vi "UHR-Fleezers Control (host) - 11.1.vi"() -> ()   [LabVIEW 2012] (continued)
            n1098 = Divide(x=w2503, y=w2487) -> (x/y=w2502:dbl[])
            n1099 = Build Array(w2522, w2521, w2536, w2520, w2519, w2533, w2488, w2504, w2489, w2486, w2502, w2487, w2500, w2499) -> (w2498:dbl[][])
            n1100 = Bundle("T1 Y", "T1 X", "T1 Sum", "T2 Y", "T2 X", "T2 Sum", "T1 FB Y", "T1 FB X", "T1 FB Sum", "T2 FB Y", "T2 FB X", "T2 FB Sum", "PSD X", "PSD Y Sum") -> (w2485:T40)  [unwired: 1 out]
            n1101 = To Word Integer(number=w2540) -> (16bit integer=w2484:i16[])
            n1102 = Cluster To Array(cluster=w2485) -> (array=w2531:string[])
          }
        }
      }
    }
    "AI labels" <- w1617
    n1103 = Decimate 1D Array(w1591) -> (w1615:void[], w1559:void[])
    n1104 = local read "DMA Update Period (s)"() -> (w1627:dbl)
    n1105 = Build Array(w1615, w1559) -> (w1693:void[])
    n1106 = local read "Data Period (s)"() -> (w1465:dbl)
    n1107 = local read "BD 1 Frequency 2 (MHz)"() -> (w1498:dbl)
    n1108 = local read "BD 1 Frequency 1 (MHz)"() -> (w1499:dbl)
    n1109 = Decimate 1D Array(w1506) -> (w1530:i16[], w1529:i16[], w1527:i16[], w1526:i16[])  [unwired: 9 out]
    n1110 = To Double Precision Float(number=w1693) -> (double precision float=w1694:dbl[])
    n1111 = local read "APD Integration Time (s)"() -> (w1572:dbl)
    n1112 = Multiply(x=w1465, y="Trap Pos. Disp. Downsample") -> (x*y=w1463:dbl)
    n1113 = Divide(x=w1530, y=w1529) -> (x/y=w1531:dbl[])
    n1114 = Divide(x=w1527, y=w1526) -> (x/y=w1528:dbl[])
    n1115 = feedback #6(0.0) -> (w1544:dbl)
    n1116 = Add(x=w1627, y=w1544) -> (x+y=w1733:dbl)
    n1117 = feedback-in #6(w1733) -> ()
    n1118 = local read "AOM X Cal (nm/MHz)"() -> (w1496:dbl)
    n1119 = To Time Stamp(1:w1544) -> (0:w1543:timestamp)
    n1120 = Split 1D Array(array=w1531, index="N El. to Ave.") -> (second subarray=w1534:dbl[])  [unwired: 1 out]
    n1121 = Split 1D Array(array=w1528, index="N El. to Ave.") -> (second subarray=w1533:dbl[])  [unwired: 1 out]
    n1122 = Multiply(x=w1465, y="Trap Disp. Downsample") -> (x*y=w1545:dbl)
    "Display Period (s)" <- w1545
    n1123 = for "Trap AI" {
      tunnel: [w2283] -> w1727 mode=indexing
      tunnel: w1543 -> [w2273]
      tunnel: "Trap Disp. Downsample" -> [w2281]
      tunnel: w1618 -> [w2279] mode=indexing
      tunnel: w1465 -> [w2278]
      tunnel: w1617 -> [w2277] mode=indexing
      tunnel: w1542 -> [w2276]
      tunnel: [w2275] -> w1583 mode=indexing
      tunnel: w1545 -> [w2274]
      workers-P: _ -> [_]
      n1124 = Bundle By Name("Y"=w2279, "dt"=w2278) -> (w2280:waveform(dbl))  [unwired: 1 out]
      n1125 = Set Waveform Attribute(5:w2277, 6:w2276, 7:w2280) -> (3:w2275:waveform(dbl))  [unwired: 1 in, 2 out]
      n1126 = call "downsample 1D array - double.vi"("Ave N"=w2281, "Array In"=w2279) -> ("Array Out"=w2282:dbl[])  [unwired: 1 out]
      n1127 = Bundle By Name(cluster=w2275, "t0"=w2273, "Y"=w2282, "dt"=w2274) -> (w2283:waveform(dbl))
    }
    n1128 = Bundle("BD 1 Frequency 1 (MHz)"=w1499, "BD 1 Frequency 2 (MHz)"=w1498) -> (w1500:T41)  [unwired: 1 out]
    n1129 = call-poly <vilib>:"Mean.vi"("X"=w1533) -> ("mean"=w1521:dbl)  [unwired: 1 out]
    n1130 = call-poly <vilib>:"Mean.vi"("X"=w1534) -> ("mean"=w1522:dbl)  [unwired: 1 out]
    n1131 = Reciprocal(x=w1545) -> (1/x=→"Trap Disp. Freq. (Hz)":dbl)
    n1132 = Cluster To Array(cluster=w1500) -> (array=w1497:dbl[])
    n1133 = local read "Trap X AI1 (DMA)"() -> (w1532:T13)
    n1134 = local read "Data points/scans (MCL)"() -> (w1705:dbl)
    n1135 = To Fixed-Point(number=w1521) -> (fixed-point=w1519:fxp<+/-,16,1>)  [unwired: 1 in]
    n1136 = To Fixed-Point(number=w1522) -> (fixed-point=w1520:fxp<+/-,16,1>)  [unwired: 1 in]
    n1137 = Bundle("Trap 1 Pos.", "Trap 2 Pos.") -> (w1541:cluster{string, string})  [unwired: 1 out]
    n1138 = Bundle By Name(cluster=w1532, "Set 1"=w1520, "Set 2"=w1519) -> (→"Trap X AI1 (DMA)":T13)
    n1139 = Cluster To Array(cluster=w1541) -> (array=w1538:string[])
    n1140 = Bundle("APD 1", "APD 2") -> (w1726:cluster{string, string})  [unwired: 1 out]
    n1141 = Select(t=-1.0, s="Negate Y Axis", f=1.0) -> (s? t:f=w1482:dbl)
    n1142 = for "Trap Position" {
      tunnel: w1547 -> [w1922] mode=indexing
      tunnel: "Trap Pos. Disp. Downsample" -> [w1921]
      tunnel: w1463 -> [w1919]
      tunnel: w1543 -> [w1918]
      tunnel: w1542 -> [w1916]
      tunnel: w1538 -> [w1915] mode=indexing
      tunnel: [w1914] -> w1452 mode=indexing
      tunnel: w1497 -> [w1912] mode=indexing
      tunnel: w1496 -> [w1910]
      tunnel: w1482 -> [w1909]
      n1143 = call "downsample 1D array - double.vi"("Ave N"=w1921, "Array In"=w1922) -> ("Array Out"=w1920:dbl[])  [unwired: 1 out]
      n1144 = Subtract(x=w1920, y=w1912) -> (x-y=w1913:dbl[])
      n1145 = Multiply(x=w1910, y=w1913) -> (x*y=w1911:dbl[])
      n1146 = Multiply(x=w1909, y=w1911) -> (x*y=w1908:dbl[])
      n1147 = Bundle By Name("Y"=w1908, "dt"=w1919, "t0"=w1918) -> (w1917:waveform(dbl))  [unwired: 1 out]
      n1148 = Set Waveform Attribute(5:w1915, 6:w1916, 7:w1917) -> (3:w1914:waveform(dbl))  [unwired: 1 in, 2 out]
    }
    n1149 = Cluster To Array(cluster=w1726) -> (array=w1723:string[])
    n1150 = for "APD" {
      tunnel: w1694 -> [w2262] mode=indexing
      tunnel: w1572 -> [w2270]
      tunnel: [w2266] -> w1579 mode=indexing
      tunnel: "APD Disp. Scale" -> [w2267]
      tunnel: w1542 -> [w2265]
      tunnel: w1723 -> [w2264] mode=indexing
      tunnel: "APD Disp. Downsample" -> [w2260]
      tunnel: [w2263] -> w1722
      workers-P: _ -> [_]
      tunnel: w1543 -> [w2259]
      n1151 = call "integrate 1D array interval - double.vi"("Ave N"=w2260, "Array In"=w2262) -> ("Array Out"=w2261:dbl[])  [unwired: 1 out]
      n1152 = Multiply(x=w2270, y=w2260) -> (x*y=w2263:dbl)
      n1153 = Divide(x=w2261, y=w2267) -> (x/y=w2268:dbl[])
      n1154 = Bundle By Name("t0"=w2259, "Y"=w2268, "dt"=w2263) -> (w2269:waveform(dbl))  [unwired: 1 out]
      n1155 = Set Waveform Attribute(5:w2264, 6:w2265, 7:w2269) -> (3:w2266:waveform(dbl))  [unwired: 1 in, 2 out]
    }
    "APD Display Period (s)" <- w1722
    n1156 = Reciprocal(x=w1722) -> (1/x=→"APD Display Freq. (Hz)":dbl)
    n1157 = local read "Display Period (s)"() -> (w1603:dbl)
    n1158 = Increment(x=w1705) -> (x+1=w1706:dbl)
    n1159 = To Double Precision Float(number=w1615) -> (double precision float=w1614:dbl[])
    n1160 = Index Array(array=w1452, index=0) -> (element=w1456:waveform(dbl))
    n1161 = Index Array(array=w1452, index=1) -> (element=w1451:waveform(dbl))
    n1162 = feedback #7(w1706) -> (w1709:dbl)
    n1163 = Select(t=0, s=w1696, f=w1709) -> (s? t:f=w1702:dbl)
    n1164 = Array Size(array=w1614) -> (size(s)=w1708:i32)
    n1165 = Add(x=w1708, y=w1702) -> (x+y=w1703:dbl)
    n1166 = Unbundle By Name(w1456) -> ("Y"=w1457:dbl[])
    n1167 = feedback #8(w1615) -> (w1692:void[])
    n1168 = Build Array (concatenate)(w1692, w1615) -> (w1689:void[])
    n1169 = feedback #9(w1559) -> (w1578:void[])
    n1170 = Divide(x="Bead Sep. Int. Time (s)", y=w1603) -> (x/y=w1492:dbl)
    n1171 = Build Array (concatenate)(w1578, w1559) -> (w1577:void[])
    n1172 = Add(x=w1457, y="FB Trap Pos Offset") -> (x+y=w1455:dbl[])
    "T1 x pos data" <- w1455
    n1173 = Greater?(x=w1703, y=w1705) -> (0:w1704:bool)
    n1174 = feedback #10(w1455) -> (w1494:dbl[])
    n1175 = Build Array (concatenate)(w1455, w1494) -> (w1493:dbl[])
    n1176 = Bundle By Name(cluster=w1456, "Y"=w1455) -> (w1454:waveform(dbl))
    n1177 = Select(t=w1702, s=w1704, f=w1703) -> (s? t:f=w1701:dbl)
    n1178 = feedback-in #7(w1701) -> ()
    n1179 = Array Size(array=w1689) -> (size(s)=w1686:i32)
    n1180 = Array Size(array=w1615) -> (size(s)=w1688:i32)
    n1181 = local read "MCL Scanning"() -> (w1699:bool)
    n1182 = local read "APD Integration Time (s)"() -> (w1586:dbl)
    n1183 = Bundle(w1454, w1451) -> (w1450:cluster{waveform(dbl), waveform(dbl)})  [unwired: 1 out]
    n1184 = Build Array (concatenate)(w1579, w1727) -> (w1581:waveform(dbl)[])
    "All Signals" <- w1581
    n1185 = Split 1D Array(array=w1493, index=w1492) -> (first subarray=w1486:dbl[])  [unwired: 1 out]
    n1186 = feedback-in #10(w1486) -> ()
    n1187 = Multiply(x=w1688, y="APD Ave N") -> (x*y=w1687:dbl)
    n1188 = Greater?(x=w1686, y=w1687) -> (0:w1690:bool)
    n1189 = Not(x=w1704) -> (.not. x?=w1698:bool)
    n1190 = Cluster To Array(cluster=w1450) -> (array=w1426:waveform(dbl)[])
    "Trap Positions" <- w1426
    n1191 = To Double Precision Float(number=w1559) -> (double precision float=w1558:dbl[])
    n1192 = call-poly <vilib>:"Mean.vi"("X"=w1486) -> ("mean"=w1485:dbl)  [unwired: 1 out]
    "Mean T1 Position (nm)" <- w1485
    n1193 = Subtract(x=w1486, y=w1485) -> (x-y=w1491:dbl[])
    n1194 = Square(x=w1491) -> (x^2=w1490:dbl[])
    n1195 = And(x=w1698, y=w1699) -> (x .and. y?=w1700:bool)
    n1196 = call-poly <vilib>:"Mean.vi"("X"=w1490) -> ("mean"=w1489:dbl)  [unwired: 1 out]
    n1197 = case shown="True" w1690 {
      tunnel: w1689 -> [w2042 w2049]
      tunnel: [w2042 w2047] -> w1632
      tunnel: w1687 -> [_ w2044]
      tunnel: w1686 -> [_ w2048]
      tunnel: w1577 -> [w2041 w2046]
      tunnel: [w2041 w2043] -> w1574
      frame False {
      }
      frame True {
        n1198 = Subtract(x=w2048, y=w2044) -> (x-y=w2045:dbl)
        n1199 = Array Subset(array=w2049, index=w2045, length=w2044) -> (w2047:void[])
        n1200 = Array Subset(array=w2046, index=w2045, length=w2044) -> (w2043:void[])
      }
    }
    n1201 = feedback-in #8(w1632) -> ()
    n1202 = feedback-in #9(w1574) -> ()
    n1203 = Square Root(x=w1489) -> (sqrt(x)=w1488:dbl)
    n1204 = Or(x=w1700, y=w1696) -> (x .or. y?=w1697:bool)
    n1205 = Equal?(x="Tab Control 6", y=T29."High Res Display") -> (x = y?=w1621:bool)
    n1206 = Multiply(x="APD Disp. Scale", y=w1579) -> (x*y=w1588:waveform(dbl)[])
    n1207 = Multiply(x=10.0, y=w1488) -> (x*y=→"Trap 1 Position RMS (A)":dbl)
    n1208 = Multiply(x="APD Disp. Downsample", y=w1586) -> (x*y=w1584:dbl)
    n1209 = Divide(x=w1588, y=w1584) -> (x/y=w1556:waveform(dbl)[])
    n1210 = case "For displaying the high resolution display (no downsampling)" shown="True" w1621 {
      tunnel: w1583 -> [_ w1942]
      frame False {
      }
      frame True {
        n1211 = Index Array(array=w1942, index="High Res. Display") -> (element=w1943:waveform(dbl))
        n1212 = call <vilib>:"Std Deviation and Variance.vi"("X"=w1943) -> ("mean"=w1950:dbl, "standard deviation"=w1955:dbl)  [unwired: 1 in, 1 out]
        "Mean Intensity" <- w1950
        "Sigma" <- w1955
        n1213 = Subtract(x=w1943, y=w1950) -> (x-y=w1949:waveform(dbl))
        n1214 = Select(t=w1949, s="Subtract mean", f=w1943) -> (s? t:f=→"1 Channel":waveform(dbl))
        n1215 = Divide(x=w1955, y=w1950) -> (x/y=→"Sigma/Mean":dbl)
        n1216 = feedback #11(1) -> (w1944:i32)
        n1217 = Greater Or Equal?(x=w1944, y="Slow mean N ave.") -> (x >= y?=w1957:bool)
        n1218 = Increment(x=w1944) -> (x+1=w1959:i32)
        n1219 = Select(t=1, s=w1957, f=w1959) -> (s? t:f=w1946:i32)
        n1220 = feedback-in #11(w1946) -> ()
        n1221 = feedback #12() -> (w1947:waveform(dbl))  [unwired: 1 out]
        n1222 = case shown="Default" w1944 {
          tunnel: [w1962 w1965] -> w1948
          tunnel: w1947 -> [w1964 _]
          tunnel: w1943 -> [w1963 w1965]
          frame Default {
            n1223 = call-poly <vilib>:"Append Waveforms.vi"("waveform B"=w1963, "waveform A"=w1964) -> ("waveform out"=w1962:waveform(dbl))  [unwired: 1 in, 8 out]
          }
          frame 1 {
          }
        }
        n1224 = feedback-in #12(w1948) -> ()
        n1225 = case shown="True" w1957 {
          tunnel: w1948 -> [_ w1961]
          frame False {
          }
          frame True {
            n1226 = call-poly <vilib>:"Mean.vi"("X"=w1961) -> ("mean"=→"Slow mean":dbl)  [unwired: 1 out]
          }
        }
      }
    }
    n1227 = Index Array(array=w1556, index=0) -> (element=w1566:waveform(dbl))
    n1228 = Index Array(array=w1556, index=1) -> (element=w1564:waveform(dbl))
    n1229 = case "For computing FFTs for display" shown="True" "Compute FFT" {
      tunnel: w1583 -> [_ w2656]
      frame False {
      }
      frame True {
        n1230 = Build Array("FFT 1 Choice 1", "FFT 1 Choice 2", "FFT 2 Choice 1", "FFT 2 Choice 2") -> (w2649:u16[])
        n1231 = Array Size(array=w2656) -> (size(s)=w2655:i32)
        n1232 = feedback-in #13(w2649) -> ()
        n1233 = feedback #13(u16[] [100, 100, 100, 100]) -> (w2650:u16[])
        n1234 = feedback-in #14("# Spectra to Ave.") -> ()
        n1235 = feedback #14("# Spectra to Ave.") -> (w2647:dbl)
        n1236 = Not Equal?(x="# Spectra to Ave.", y=w2647) -> (x != y?=w2646:bool)
        n1237 = Not Equal?(x=w2649, y=w2650) -> (x != y?=w2648:bool)
        n1238 = feedback #15(1.0) -> (w2633:dbl)
        n1239 = Compound Arithmetic op=OR("Reset FFT", w2648, w2646) -> (w2631:bool)
        n1240 = Select(t=1.0, s=w2631, f=w2633) -> (s? t:f=w2635:dbl)
        n1241 = Greater?(x=w2635, y="# Spectra to Ave.") -> (0:w2654:bool)
        n1242 = Increment(x=w2635) -> (x+1=w2634:dbl)
        n1243 = feedback-in #15(w2634) -> ()
        n1244 = local read "DMA Update Period (s)"() -> (w2629:dbl)
        n1245 = Multiply(x="# Spectra to Ave.", y=w2629) -> (x*y=→"Ave. Time (s)":dbl)
        n1246 = Build Array(cluster{"f0":dbl, "df":dbl, "magnitude":dbl[]} {"f0"=0.0, "df"=0.0, "magnitude"=[]} ("PSD")) -> (w2638:cluster{"f0":dbl, "df":dbl, "magnitude":dbl[]}[])
        n1247 = Build Array(w2638, w2638, w2638, w2638) -> (w2640:T42)
        n1248 = feedback #16(w2640) -> (w2645:T42)
        n1249 = for {
          N: 4 -> [_]
          tunnel: w2649 -> [w2678] mode=indexing
          tunnel: w2656 -> [w2679]
          tunnel: w2655 -> [w2681]
          tunnel: w2631 -> [w2674]
          tunnel: w2654 -> [w2673]
          tunnel: "# Spectra to Ave." -> [w2672]
          tunnel: [w2671] -> w2644 mode=indexing
          tunnel: w2645 -> [w2676] mode=indexing
          tunnel: [w2675] -> w2632 mode=indexing
          tunnel: w2635 -> [w2670]
          n1250 = Less?(x=w2678, y=w2681) -> (x < y?=w2680:bool)
          n1251 = Index Array(array=w2679, index=w2678) -> (element=w2677:waveform(dbl))
          n1252 = case shown="True" w2680 {
            tunnel: w2677 -> [_ w2698]
            tunnel: w2676 -> [w2683 w2696]
            tunnel: [w2683 w2684] -> w2675
            tunnel: w2674 -> [_ w2695]
            tunnel: w2673 -> [_ w2688]
            tunnel: w2672 -> [_ w2687]
            tunnel: [cluster{"f0":dbl, "df":dbl, "magnitude":dbl[]} {"f0"=0.0, "df"=0.0, "magnitude"=[]} ("PSD") w2689] -> w2671
            tunnel: w2670 -> [_ w2686]
            frame False {
            }
            frame True {
              n1253 = call <vilib>:"Std Deviation and Variance.vi"("X"=w2698) -> ("mean"=w2699:dbl)  [unwired: 1 in, 2 out]
              n1254 = Subtract(x=w2698, y=w2699) -> (x-y=w2697:waveform(dbl))
              n1255 = xnode "Spectral Measurements"("Signals"=w2697) -> ("PSD"=w2691:cluster{"f0":dbl, "df":dbl, "magnitude":dbl[]})  [unwired: 1 in, 1 out]
              n1256 = case shown="False" w2695 {
                tunnel: w2696 -> [w2708 _]
                tunnel: [w2704 w2713] -> w2684
                tunnel: w2691 -> [w2707 w2714]
                tunnel: w2688 -> [w2706 _]
                frame False {
                  n1257 = Build Array (concatenate)(w2708, w2707) -> (w2705:cluster{"f0":dbl, "df":dbl, "magnitude":dbl[]}[])
                  n1258 = case shown="True" w2706 {
                    tunnel: w2705 -> [w2709 w2712]
                    tunnel: [w2709 w2710] -> w2704
                    frame False {
                    }
                    frame True {
                      n1259 = Delete From Array(array=w2712, index=0) -> (array with subset deleted=w2710:cluster{"f0":dbl, "df":dbl, "magnitude":dbl[]}[])  [unwired: 1 in, 1 out]
                    }
                  }
                }
                frame True {
                  n1260 = Build Array(w2714) -> (w2713:cluster{"f0":dbl, "df":dbl, "magnitude":dbl[]}[])
                }
              }
              n1261 = for {
                tunnel: w2684 -> [w2703] mode=indexing
                tunnel: [w2702] -> w2694 mode=indexing
                workers-P: _ -> [_]
                n1262 = Unbundle By Name(w2703) -> ("magnitude"=w2702:dbl[])
              }
              n1263 = Transpose 2D Array(2D array=w2694) -> (transposed array=w2693:dbl[][])
              n1264 = for {
                tunnel: w2693 -> [w2701] mode=indexing
                tunnel: [w2700] -> w2692 mode=indexing
                workers-P: _ -> [_]
                n1265 = Add Array Elements(numeric array=w2701) -> (sum=w2700:dbl)
              }
              n1266 = Select(t=w2687, s=w2688, f=w2686) -> (s? t:f=w2685:dbl)
              n1267 = Divide(x=w2692, y=w2685) -> (x/y=w2690:dbl[])
              n1268 = Bundle By Name(cluster=w2691, "magnitude"=w2690) -> (w2689:cluster{"f0":dbl, "df":dbl, "magnitude":dbl[]})
            }
          }
        }
        n1269 = case shown="True" w2631 {
          tunnel: w2632 -> [w2663 w2669]
          tunnel: [w2663 w2664] -> w2630
          frame False {
          }
          frame True {
            n1270 = Array Subset(array=w2669, index (row)=0 ("index"), length (row)=4 ("length"), index (col)=0 ("index"), length (col)=1 ("length")) -> (w2664:T42)
          }
        }
        n1271 = feedback-in #16(w2630) -> ()
        n1272 = Split 1D Array(array=w2644, index=2) -> (first subarray=→"FFT 1":cluster{"f0":dbl, "df":dbl, "magnitude":dbl[]}[], second subarray=→"FFT 2":cluster{"f0":dbl, "df":dbl, "magnitude":dbl[]}[])
      }
    }
    n1273 = case "For plotting results of scanning MCL" shown="True" w1697 {
      tunnel: w1696 -> [_ w2082]
      tunnel: w1614 -> [_ w2178]
      tunnel: w1705 -> [_ _]
      tunnel: w1583 -> [_ w2152]
      tunnel: w1558 -> [_ w2083]
      tunnel: w1557 -> [_ w2056]
      frame False {
      }
      frame True {
        w2063 = u32 0 items=["Horizontal", "Vertical", "Central", "1st Diagonal", "2nd Diagonal"] ("Type of Symmetry")
        w2091 = u32 0 items=["Horizontal", "Vertical", "Central", "1st Diagonal", "2nd Diagonal"] ("Type of Symmetry")
        w2094 = u32 0 items=["Horizontal", "Vertical", "Central", "1st Diagonal", "2nd Diagonal"] ("Type of Symmetry")
        w2123 = u32 0 items=["Horizontal", "Vertical", "Central", "1st Diagonal", "2nd Diagonal"] ("Type of Symmetry")
        n1274 = Index Array(array=w2152, index=10) -> (element=w2158:waveform(dbl))
        n1275 = Index Array(array=w2152, index=11) -> (element=w2155:waveform(dbl))
        n1276 = local read "Cycles/step (MCL)"() -> (w2108:u64)
        n1277 = Index Array(array=w2152, index="Channel") -> (element=w2154:waveform(dbl))
        n1278 = Unbundle(w2056) -> ("New Image"=w2055:T2, "New Image"=w2054:T2, "New Image"=w2053:T2, "New Image"=w2052:T2)
        n1279 = Unbundle By Name(w2158) -> ("Y"=w2110:dbl[])
        n1280 = Unbundle By Name(w2155) -> ("Y"=w2112:dbl[])
        n1281 = Unbundle By Name(w2154) -> ("Y"=w2117:dbl[])
        n1282 = call "downsample 1D array - double.vi"("Ave N"=w2108, "Array In"=w2110) -> ("Array Out"=w2109:dbl[])  [unwired: 1 out]
        n1283 = call "downsample 1D array - double.vi"("Ave N"=w2108, "Array In"=w2112) -> ("Array Out"=w2111:dbl[])  [unwired: 1 out]
        n1284 = call "downsample 1D array - double.vi"("Ave N"=w2108, "Array In"=w2117) -> ("Array Out"=w2116:dbl[])  [unwired: 1 out]
        n1285 = feedback #17(w2178) -> (w2179:dbl[])
        n1286 = Build Array (concatenate)(w2179, w2178) -> (w2160:dbl[])
        n1287 = feedback #18(w2083) -> (w2085:dbl[])
        n1288 = Build Array (concatenate)(w2085, w2083) -> (w2084:dbl[])
        n1289 = local read "Scan steps (MCL)"() -> (w2065:u64)
        n1290 = Select(t=w2178, s=w2082, f=w2160) -> (s? t:f=w2164:dbl[])
        n1291 = feedback-in #17(w2164) -> ()
        n1292 = Select(t=w2083, s=w2082, f=w2084) -> (s? t:f=w2066:dbl[])
        n1293 = feedback-in #18(w2066) -> ()
        n1294 = local read "Scan lines (y)"() -> (w2051:u64)
        n1295 = local read "N APD Samp/step"() -> (w2067:dbl)
        n1296 = feedback #19(w2109) -> (w2166:dbl[])
        n1297 = Build Array (concatenate)(w2166, w2109) -> (w2157:dbl[])
        n1298 = feedback #20(w2116) -> (w2176:dbl[])
        n1299 = Build Array (concatenate)(w2176, w2116) -> (w2175:dbl[])
        n1300 = feedback #21(w2111) -> (w2168:dbl[])
        n1301 = Build Array (concatenate)(w2168, w2111) -> (w2169:dbl[])
        n1302 = Select(t=w2109, s=w2082, f=w2157) -> (s? t:f=w2113:dbl[])
        n1303 = feedback-in #19(w2113) -> ()
        n1304 = Select(t=w2116, s=w2082, f=w2175) -> (s? t:f=w2115:dbl[])
        n1305 = feedback-in #20(w2115) -> ()
        n1306 = Select(t=w2111, s=w2082, f=w2169) -> (s? t:f=w2114:dbl[])
        n1307 = feedback-in #21(w2114) -> ()
        n1308 = Multiply(x=w2065, y=u64 2) -> (x*y=w2050:u64)
        n1309 = call "integrate 1D array interval - double.vi"("Ave N"=w2067, "Array In"=w2066) -> ("Array Out"=w2078:dbl[])  [unwired: 1 out]
        n1310 = call "integrate 1D array interval - double.vi"("Ave N"=w2067, "Array In"=w2164) -> ("Array Out"=w2163:dbl[])  [unwired: 1 out]
        n1311 = Array Size(array=w2078) -> (size(s)=w2079:i32)
        n1312 = Array Size(array=w2163) -> (size(s)=w2165:i32)
        n1313 = Multiply(x=w2051, y=w2050) -> (x*y=w2081:u64)
        n1314 = Multiply(x=w2051, y=w2050) -> (x*y=w2173:u64)
        n1315 = call-poly <vilib>:"Mean.vi"("X"=w2113) -> ("mean"=w2097:dbl)  [unwired: 1 out]
        n1316 = Subtract(x=w2081, y=w2079) -> (x-y=w2072:u64)
        n1317 = call-poly <vilib>:"Mean.vi"("X"=w2115) -> ("mean"=w2102:dbl)  [unwired: 1 out]
        n1318 = call-poly <vilib>:"Mean.vi"("X"=w2114) -> ("mean"=w2100:dbl)  [unwired: 1 out]
        n1319 = call-poly <vilib>:"Mean.vi"("X"=w2078) -> ("mean"=w2069:dbl)  [unwired: 1 out]
        n1320 = Subtract(x=w2173, y=w2165) -> (x-y=w2107:u64)
        n1321 = call-poly <vilib>:"Mean.vi"("X"=w2163) -> ("mean"=w2104:dbl)  [unwired: 1 out]
        n1322 = Initialize Array(1.0 ("element"), w2072) -> (w2068:dbl[])
        n1323 = Initialize Array(1.0 ("element"), w2107) -> (w2098:dbl[])
        n1324 = Multiply(x=w2068, y=w2069) -> (x*y=w2070:dbl[])
        n1325 = Multiply(x=w2098, y=w2100) -> (x*y=w2101:dbl[])
        n1326 = Multiply(x=w2098, y=w2102) -> (x*y=w2103:dbl[])
        n1327 = Multiply(x=w2098, y=w2097) -> (x*y=w2099:dbl[])
        n1328 = Multiply(x=w2098, y=w2104) -> (x*y=w2105:dbl[])
        n1329 = Build Array (concatenate)(w2113, w2099) -> (w2167:dbl[])
        n1330 = Build Array (concatenate)(w2115, w2103) -> (w2171:dbl[])
        n1331 = Build Array (concatenate)(w2114, w2101) -> (w2170:dbl[])
        n1332 = Build Array (concatenate)(w2078, w2070) -> (w2080:dbl[])
        n1333 = Build Array (concatenate)(w2163, w2105) -> (w2172:dbl[])
        n1334 = Reshape Array(w2167, w2051, w2050) -> (w2133:dbl[][])
        n1335 = Reshape Array(w2080, w2051, w2050) -> (w2076:dbl[][])
        n1336 = Reshape Array(w2171, w2051, w2050) -> (w2125:dbl[][])
        n1337 = Reshape Array(w2170, w2051, w2050) -> (w2140:dbl[][])
        n1338 = Reshape Array(w2172, w2051, w2050) -> (w2150:dbl[][])
        n1339 = Array Subset(array=w2140, index (col)=0 ("index"), length (col)=w2065) -> (w2145:dbl[][])  [unwired: 2 in]
        n1340 = Array Subset(array=w2140, index (col)=w2065) -> (w2143:dbl[][])  [unwired: 3 in]
        n1341 = Array Subset(array=w2125, index (col)=0 ("index"), length (col)=w2065) -> (w2131:dbl[][])  [unwired: 2 in]
        n1342 = Array Subset(array=w2125, index (col)=w2065) -> (w2129:dbl[][])  [unwired: 3 in]
        n1343 = Array Subset(array=w2076, index (col)=0 ("index"), length (col)=w2065) -> (w2075:dbl[][])  [unwired: 2 in]
        n1344 = Array Subset(array=w2076, index (col)=w2065) -> (w2073:dbl[][])  [unwired: 3 in]
        n1345 = Array Subset(array=w2150, index (col)=0 ("index"), length (col)=w2065) -> (w2149:dbl[][])  [unwired: 2 in]
        n1346 = Array Subset(array=w2150, index (col)=w2065) -> (w2147:dbl[][])  [unwired: 3 in]
        n1347 = Array Subset(array=w2133, index (col)=0 ("index"), length (col)=w2065) -> (w2138:dbl[][])  [unwired: 2 in]
        n1348 = Array Subset(array=w2133, index (col)=w2065) -> (w2136:dbl[][])  [unwired: 3 in]
        n1349 = for {
          tunnel: w2145 -> [w2187] mode=indexing
          tunnel: [w2186] -> w2144 mode=indexing
          workers-P: _ -> [_]
          n1350 = Reverse 1D Array(array=w2187) -> (reversed array=w2186:dbl[])
        }
        n1351 = for {
          tunnel: w2131 -> [w2183] mode=indexing
          tunnel: [w2182] -> w2130 mode=indexing
          workers-P: _ -> [_]
          n1352 = Reverse 1D Array(array=w2183) -> (reversed array=w2182:dbl[])
        }
        n1353 = for {
          tunnel: w2075 -> [w2181] mode=indexing
          tunnel: [w2180] -> w2074 mode=indexing
          workers-P: _ -> [_]
          n1354 = Reverse 1D Array(array=w2181) -> (reversed array=w2180:dbl[])
        }
        n1355 = for {
          tunnel: w2149 -> [w2189] mode=indexing
          tunnel: [w2188] -> w2148 mode=indexing
          workers-P: _ -> [_]
          n1356 = Reverse 1D Array(array=w2189) -> (reversed array=w2188:dbl[])
        }
        n1357 = for {
          tunnel: w2138 -> [w2185] mode=indexing
          tunnel: [w2184] -> w2137 mode=indexing
          workers-P: _ -> [_]
          n1358 = Reverse 1D Array(array=w2185) -> (reversed array=w2184:dbl[])
        }
        n1359 = Index Array(array=w2150, index (row)=0) -> (element=→"Waveform Graph":dbl[])  [unwired: 1 in]
        n1360 = Add(x=w2144, y=w2143) -> (x+y=w2142:dbl[][])
        n1361 = Add(x=w2130, y=w2129) -> (x+y=w2128:dbl[][])
        n1362 = Add(x=w2074, y=w2073) -> (x+y=w2058:dbl[][])
        n1363 = Add(x=w2148, y=w2147) -> (x+y=w2122:dbl[][])
        n1364 = Add(x=w2137, y=w2136) -> (x+y=w2135:dbl[][])
        n1365 = Divide(x=w2128, y=2) -> (x/y=w2126:dbl[][])
        n1366 = Divide(x=w2142, y=2) -> (x/y=w2087:dbl[][])
        n1367 = Divide(x=w2135, y=2) -> (x/y=w2089:dbl[][])
        n1368 = To Single Precision Float(number=w2122) -> (single precision float=w2121:sgl[][])
        n1369 = Transpose 2D Array(2D array=w2126) -> (transposed array=→"Data map":dbl[][])
        n1370 = To Single Precision Float(number=w2058) -> (single precision float=w2062:sgl[][])
        n1371 = To Single Precision Float(number=w2087) -> (single precision float=w2093:sgl[][])
        n1372 = To Single Precision Float(number=w2089) -> (single precision float=w2090:sgl[][])
        n1373 = call "IMAQ ArrayToImage"("Image Pixels (Float)"=w2121, "Image"=w2055) -> ("Image Out"=w2124:T2)  [unwired: 8 in, 1 out]
        n1374 = call "IMAQ ArrayToImage"("Image Pixels (Float)"=w2062, "Image"=w2054) -> ("Image Out"=w2064:T2)  [unwired: 8 in, 1 out]
        n1375 = call "IMAQ ArrayToImage"("Image Pixels (Float)"=w2093, "Image"=w2053) -> ("Image Out"=w2095:T2)  [unwired: 8 in, 1 out]
        n1376 = call "IMAQ ArrayToImage"("Image Pixels (Float)"=w2090, "Image"=w2052) -> ("Image Out"=w2092:T2)  [unwired: 8 in, 1 out]
        n1377 = call "IMAQ Symmetry"("Type of Symmetry"=w2123, "Image Src"=w2124) -> ("Image Dst Out"=w2119:T2)  [unwired: 3 in, 1 out]
        n1378 = call "IMAQ Symmetry"("Type of Symmetry"=w2063, "Image Src"=w2064) -> ("Image Dst Out"=w2060:T2)  [unwired: 3 in, 1 out]
        n1379 = call "IMAQ Symmetry"("Type of Symmetry"=w2094, "Image Src"=w2095) -> ("Image Dst Out"=→"Detection Laser X":T2)  [unwired: 3 in, 1 out]
        n1380 = call "IMAQ Symmetry"("Type of Symmetry"=w2091, "Image Src"=w2092) -> ("Image Dst Out"=→"Detection Laser Y":T2)  [unwired: 3 in, 1 out]
        n1381 = call "IMAQ Set Simple Calibration"("Calibration Axis Info"=T30 {"Origin Pixel"={"X"=0.0, "Y"=0.0}, "Angle Relative to Horizontal (deg)"=0.0, "Axis Reference"=0}, "Grid Descriptor"=T31 {"X Step"=0.3, "Y Step"=0.3, "Unit"=enum."Undefined"}, "Image"=w2119) -> ("Calibrated Image"=→"APD 1":T2)  [unwired: 7 in, 1 out]
        n1382 = call "IMAQ Set Simple Calibration"("Calibration Axis Info"=T30 {"Origin Pixel"={"X"=0.0, "Y"=0.0}, "Angle Relative to Horizontal (deg)"=0.0, "Axis Reference"=0}, "Grid Descriptor"=T31 {"X Step"=0.3, "Y Step"=0.3, "Unit"=enum."Undefined"}, "Image"=w2060) -> ("Calibrated Image"=→"APD 2":T2)  [unwired: 7 in, 1 out]
      }
    }
    n1383 = Subtract(x=w1564, y="APD 2 Offset") -> (x-y=w1561:waveform(dbl))
    n1384 = Subtract(x=w1566, y="APD 1 Offset") -> (x-y=w1562:waveform(dbl))
    n1385 = Index Array(array=w1581, index=3) -> (element=w1641:waveform(dbl))
    n1386 = Index Array(array=w1581, index=6) -> (element=w1638:waveform(dbl))
    n1387 = Build Array(w1562, w1561) -> (→"APD Chart":waveform(dbl)[])
    n1388 = Array Size(array=w1632) -> (size(s)=w1685:i32)
    n1389 = call <vilib>:"Std Deviation and Variance.vi"("X"=w1574) -> ("standard deviation"=w1573:dbl)  [unwired: 1 in, 2 out]
    n1390 = Add Array Elements(numeric array=w1574) -> (sum=w1576:dbl)
    n1391 = Add Array Elements(numeric array=w1632) -> (sum=w1695:dbl)
    n1392 = call <vilib>:"Std Deviation and Variance.vi"("X"=w1632) -> ("standard deviation"=w1631:dbl)  [unwired: 1 in, 2 out]
    n1393 = Divide(x="T1 offset_x (mV)", y=1000.0) -> (x/y=w1642:dbl)
    n1394 = Divide(x=w1573, y=w1572) -> (x/y=w1569:dbl)
    "Rate sigma (Hz) 2" <- w1569
    n1395 = Multiply(x=w1572, y=w1685) -> (x*y=w1575:dbl)
    "Int. Time (s)" <- w1575
    n1396 = Divide(x=w1576, y=w1575) -> (x/y=w1570:dbl)
    "APD 2 Rate (Hz)" <- w1570
    n1397 = Divide(x=w1695, y=w1575) -> (x/y=w1629:dbl)
    "APD 1 Rate (Hz)" <- w1629
    n1398 = Divide(x=w1631, y=w1572) -> (x/y=w1630:dbl)
    "Rate sigma (Hz)" <- w1630
    n1399 = Divide(x=w1569, y=w1570) -> (x/y=→"Sigma/Mean 2":dbl)
    n1400 = Divide(x=w1630, y=w1629) -> (x/y=→"Sigma/Mean":dbl)
    n1401 = feedback-in #22("Calibration") -> ()
    n1402 = feedback #22(u16 1 ("Calibration")) -> (w1662:u16)
    n1403 = Divide(x="T2 offset_x (mV)", y=1000.0) -> (x/y=w1640:dbl)
    n1404 = case shown="0, Default" "Calibration" {
      tunnel: "T1 alpha_x (nm/V)" -> [_ w2018 w2039]
      tunnel: "T1 kappa_x (pN/nm)" -> [_ _ w2029]
      tunnel: "T2 alpha_x (nm/V)" -> [_ w2017 w2037]
      tunnel: "T2 kappa_x (pN/nm)" -> [_ _ w2030]
      tunnel: w1641 -> [w2000 w2015 w2035]
      tunnel: w1638 -> [w1999 w2013 w2033]
      tunnel: [w2000 w2012 w2032] -> w1671
      tunnel: [w1999 w2011 w2031] -> w1670
      tunnel: ["T1 X (V)" ("Label.Text") "T1 X (nm)" ("Label.Text") "T1 X (pN)" ("Label.Text")] -> w1659
      tunnel: ["T2 X (V)" ("Label.Text") "T2 X (nm)" ("Label.Text") "T2 X (pN)" ("Label.Text")] -> w1658
      tunnel: ["Position (V)" ("Label.Text") "Position (nm)" ("Label.Text") "Force (pN)" ("Label.Text")] -> w1660
      tunnel: w1640 -> [_ w2003 w2022]
      tunnel: w1642 -> [_ w2006 w2024]
      tunnel: ["Mean (V)" ("Label.Text") "Mean (nm)" ("Label.Text") "Mean (pN)" ("Label.Text")] -> w1655
      tunnel: ["Difference (V)" ("Label.Text") "Difference (nm)" ("Label.Text") "Difference (pN)" ("Label.Text")] -> w1589
      frame 0, Default {
      }
      frame 1 {
        n1405 = Unbundle By Name(w2015) -> ("Y"=w2019:dbl[])
        n1406 = Unbundle By Name(w2013) -> ("Y"=w2004:dbl[])
        n1407 = Subtract(x=w2019, y=w2006) -> (x-y=w2007:dbl[])
        n1408 = Subtract(x=w2004, y=w2003) -> (x-y=w2005:dbl[])
        n1409 = Multiply(x=w2005, y=w2017) -> (x*y=w2014:dbl[])
        n1410 = Multiply(x=w2018, y=w2007) -> (x*y=w2016:dbl[])
        n1411 = Bundle By Name(cluster=w2013, "Y"=w2014) -> (w2011:waveform(dbl))
        n1412 = Bundle By Name(cluster=w2015, "Y"=w2016) -> (w2012:waveform(dbl))
      }
      frame 2 {
        n1413 = Unbundle By Name(w2035) -> ("Y"=w2040:dbl[])
        n1414 = Unbundle By Name(w2033) -> ("Y"=w2038:dbl[])
        n1415 = Subtract(x=w2038, y=w2022) -> (x-y=w2023:dbl[])
        n1416 = Subtract(x=w2040, y=w2024) -> (x-y=w2025:dbl[])
        n1417 = Compound Arithmetic op=MULTIPLY(w2023, w2037, w2030) -> (w2034:dbl[])
        n1418 = Compound Arithmetic op=MULTIPLY(w2029, w2039, w2025) -> (w2036:dbl[])
        n1419 = Bundle By Name(cluster=w2033, "Y"=w2034) -> (w2031:waveform(dbl))
        n1420 = Bundle By Name(cluster=w2035, "Y"=w2036) -> (w2032:waveform(dbl))
      }
    }
    n1421 = Not Equal?(x=w1662, y="Calibration") -> (x != y?=w1619:bool)
    n1422 = case shown="True" w1619 {
      tunnel: w1660 -> [_ w1993]
      tunnel: w1659 -> [_ w1992]
      tunnel: w1658 -> [_ w1991]
      tunnel: w1655 -> [_ w1990]
      tunnel: w1589 -> [_ w1989]
      frame False {
      }
      frame True {
        n1423 = property on="Force" class="WFChart (strict)"("YScale.NameLbl.Text"=w1993) -> ()  [unwired: 2 in, 2 out]
        n1424 = property on="T2 X" class="DigNum (strict)"("Caption.Text"=w1991) -> ()  [unwired: 2 in, 2 out]
        n1425 = property on="T1 X" class="DigNum (strict)"("Caption.Text"=w1992) -> ()  [unwired: 2 in, 2 out]
        n1426 = property on="Mean" class="DigNum (strict)"("Caption.Text"=w1990) -> ()  [unwired: 2 in, 2 out]
        n1427 = property on="Difference" class="DigNum (strict)"("Caption.Text"=w1989) -> ()  [unwired: 2 in, 2 out]
      }
    }
    n1428 = Unbundle By Name(w1641) -> ("Y"=w1644:dbl[])
    n1429 = Unbundle By Name(w1638) -> ("Y"=w1647:dbl[])
    n1430 = Subtract(x=w1644, y=w1642) -> (x-y=w1645:dbl[])
    n1431 = Subtract(x=w1647, y=w1640) -> (x-y=w1646:dbl[])
    n1432 = Multiply(x=w1646, y="T2 alpha_x (nm/V)") -> (x*y=w1431:dbl[])
    n1433 = Multiply(x="T1 alpha_x (nm/V)", y=w1645) -> (x*y=w1432:dbl[])
    n1434 = Not(x="Trap Trig. Fl.") -> (.not. x?=w1468:bool)
    n1435 = Multiply(x=w1670, y=-1.0) -> (x*y=w1649:waveform(dbl))
    n1436 = Subtract(x=w1432, y=w1431) -> (x-y=w1637:dbl[])
    n1437 = Unbundle By Name(w1670) -> ("Y"=w1608:dbl[])
    n1438 = Unbundle By Name(w1671) -> ("Y"=w1433:dbl[])
    n1439 = Negate(x=w1637) -> (-x=w1429:dbl[])
    n1440 = Build Array(w1671, w1649) -> (→"Force":waveform(dbl)[])
    n1441 = Subtract(x=w1429, y="Offset (nm)") -> (x-y=w1606:dbl[])
    n1442 = case shown="True" "Read Lateness and Rel Phase" {
      tunnel: w1449 -> [w1966 w1988]
      tunnel: w1448 -> [w1967 w1987]
      tunnel: [w1966 w1986] -> w1635
      tunnel: [w1967 w1985] -> w1634
      frame False {
      }
      frame True {
        n1443 = xnode "Read/Write Control"("FPGA VI Reference In"=w1988, "error in"=w1987) -> ("FPGA VI Reference Out"=w1986:T19, "error out"=w1985:errorcluster, "GI Relative phase"=→"GI relative phase":i16, "Relative phase"=→"Relative phase (AI1)":i16, "AI Late Counter"=→"Late Counter (AI1)":u16, "GI Late Counter"=→"GI Late Counter":u16, "MCL Late Counter"=→"MCL Late Counter":u16, "MCL Relative Phase"=→"Relative Phase (MCL)":i16, "APD Acq Relative Phase"=→"APD Acq Relative Phase":i16, "APD 1 Gate Relative Phase"=→"APD 1 Gate Relative Phase":i16, "APD 2 Gate Relative Phase"=→"APD 2 Gate Relative Phase":i16, "APD Acq Late Counter"=→"APD Acq Late Counter":u16, "APD 1 Gate Late Counter"=→"APD 1 Gate Late Counter":u16, "APD 2 Gate Late Counter"=→"APD 2 Gate Late Counter":u16, "Green FB Relative Phase"=→"Relative phase (Green FB)":i16, "GI Relative phase 2"=→"GI relative phase 2":i16, "GI Late Counter 2"=→"GI Late Counter 2":u16, "Trap Pos FIFO Timeout"=→"Trap Pos FIFO Timeout":u16, "Trap AI FIFO Timeout"=→"Trap AI FIFO Timeout":u16)
      }
    }
    n1444 = call-poly <vilib>:"Mean.vi"("X"=w1608) -> ("mean"=w1435:dbl)  [unwired: 1 out]
    "T2 X" <- w1435
    n1445 = Negate(x=w1608) -> (-x=w1609:dbl[])
    n1446 = call-poly <vilib>:"Mean.vi"("X"=w1433) -> ("mean"=w1436:dbl)  [unwired: 1 out]
    "T1 X" <- w1436
    n1447 = Negate(x=w1435) -> (-x=w1434:dbl)
    n1448 = Bundle By Name(cluster=w1641, "Y"=w1606) -> (w1580:waveform(dbl))
    "Bead Separation" <- w1580
    n1449 = Add(x=w1433, y=w1609) -> (x+y=w1610:dbl[])
    n1450 = Add(x=w1436, y=w1434) -> (x+y=w1657:dbl)
    n1451 = Subtract(x=w1436, y=w1434) -> (x-y=→"Difference":dbl)
    n1452 = Divide(x=w1610, y=2.0) -> (x/y=→"Vec Mean of T1 T2":dbl[])
    n1453 = Divide(x=w1657, y=2.0) -> (x/y=w1612:dbl)
    "Mean" <- w1612
    n1454 = feedback-in #23("Trap Trig. Fl.") -> ()
    n1455 = feedback #23("Trap Trig. Fl.") -> (w1466:bool)
    n1456 = And(x=w1468, y=w1466) -> (x .and. y?=w1467:bool)
    n1457 = case "If have just turned off triggering" shown="True" w1467 {
      tunnel: w1449 -> [_ w1801]
      tunnel: w1448 -> [_ w1800]
      frame False {
      }
      frame True {
        w1799 = FALSE ("FPGA Trap Trig")
        n1458 = xnode "Read/Write Control"("FPGA VI Reference In"=w1801, "error in"=w1800, "FPGA Trap Trig"=w1799) -> ("FPGA VI Reference Out"=w1798:T19, "error out"=w1797:errorcluster)
        n1459 = xnode "Read/Write Control"("FPGA VI Reference In"=w1798, "error in"=w1797, "TTrig?"=w1799) -> ()  [unwired: 2 out]
        n1460 = local write "Initializing"(FALSE ("Initializing")) -> ()
        n1461 = local write "Triggered"(FALSE ("Triggered")) -> ()
        n1462 = local write "Waiting"(FALSE ("Waiting")) -> ()
      }
    }
    n1463 = Not(x=w1466) -> (.not. x?=w1479:bool)
    n1464 = And(x="Trap Trig. Fl.", y=w1479) -> (x .and. y?=w1476:bool)
    n1465 = local read "Tether"() -> (w1613:bool)
    n1466 = Or(x=w1476, y="Reinitialize") -> (x .or. y?=w1462:bool)
    n1467 = feedback #24(w1472) -> (w1477:string)
    n1468 = Select(t=w1472, s=w1476, f=w1477) -> (s? t:f=w1471:string)
    n1469 = Select(t=w1472, s="Reinitialize", f=w1471) -> (s? t:f=w1470:string)
    n1470 = feedback #25(0) -> (w1474:i32)
    n1471 = feedback #26(w1606) -> (w1605:dbl[])
    n1472 = Build Array (concatenate)(w1606, w1605) -> (w1430:dbl[])
    n1473 = case "For determining if there is a tether still" shown="True" w1613 {
      tunnel: w1612 -> [_ w1925]
      frame False {
      }
      frame True {
        n1474 = Greater?(x="Lost Tether Alarm Threshold (pN)", y=w1925) -> (0:w1923:bool)
        n1475 = case shown="True" w1923 {
          frame False {
          }
          frame True {
            w1926 = FALSE ("Value (Signaling)")
            n1476 = flat-sequence {
              frame #0 {
                # "stop only if saving"
                n1477 = local read "Saving..."() -> (w1938:bool)
                n1478 = And(x=w1938, y="TA Cancel Save?") -> (x .and. y?=w1937:bool)
                n1479 = local write "Stop Saving"(w1937) -> ()
              }
              frame #1 {
                n1480 = case shown="True" "TA Green Off?" {
                  frame False {
                  }
                  frame True {
                    w1941 = FALSE ("Fl. Triggered...")
                    n1481 = local write "Fl. Triggered..."(w1941) -> ()
                    n1482 = property on="Green Laser ON/Interlacing" class="Bool (strict)"("Val(Sgnl)"=w1941) -> ()  [unwired: 2 in, 2 out]
                  }
                }
              }
            }
            n1483 = local read "Time tether formed"() -> (w1932:timestamp)
            n1484 = Get Date/Time In Seconds() -> (seconds since 1Jan1904=w1933:timestamp)
            n1485 = Subtract(x=w1933, y=w1932) -> (x-y=w1931:dbl)
            n1486 = Number To Decimal String(number=w1931) -> (decimal integer string=w1928:string)  [unwired: 1 out]
            n1487 = local read "Messages"() -> (w1935:string)
            n1488 = call <vilib>:"Beep.vi"() -> ()  [unwired: 3 in, 9 out]
            n1489 = Concatenate Strings("Lost tether (" ("Message to add"), w1928, " s)." ("string")) -> (w1930:string)
            n1490 = local write "Tether"(FALSE ("Tether")) -> ()
            n1491 = call "Update messages.vi"("Message to add"=w1930, "Old message string"=w1935) -> ("New message string"=w1934:string)
            n1492 = local write "Messages"(w1934) -> ()
            n1493 = property on="Fl. Triggered..." class="Bool (strict)"("Val(Sgnl)"=w1926) -> ()  [unwired: 2 in, 2 out]
            n1494 = local write "Dip for Protein"(w1926) -> ()
            n1495 = property on="Trap Pos. FB ON" class="Bool (strict)"("Val(Sgnl)"=w1926) -> ()  [unwired: 2 in, 2 out]
            n1496 = property on="Trap Trig. Fl." class="Bool (strict)"("Val(Sgnl)"=w1926) -> ()  [unwired: 2 in, 2 out]
          }
        }
      }
    }
    n1497 = case "For triggering actions based on the trap position (e.g., turning the excitation laser on if trap under feedback moves so far)" shown="True" "Trap Trig. Fl." {
      tunnel: w1457 -> [_ w1814]
      tunnel: w1470 -> [_ w1813]
      tunnel: ["" ("t") w1812] -> w1478
      tunnel: w1462 -> [_ w1811]
      tunnel: [0 ("t") w1810] -> w1475
      tunnel: w1474 -> [_ w1809]
      tunnel: w1449 -> [_ w1808]
      tunnel: w1448 -> [_ w1807]
      frame False {
      }
      frame True {
        n1498 = case shown="\"Wait for trigger\"" w1813 {
          tunnel: w1814 -> [w1831 _ _ w1879]
          tunnel: [w1828 w1860 "" ("t") w1882] -> w1812
          tunnel: w1811 -> [_ _ _ w1870]
          tunnel: [w1827 w1857 0 ("t") w1871] -> w1810
          tunnel: w1809 -> [_ w1859 _ w1877]
          tunnel: w1808 -> [w1816 w1854 _ w1873]
          tunnel: w1807 -> [w1815 w1853 _ w1872]
          frame "Wait for trigger" {
            n1499 = local read "Trap Trig. (FPGA)"() -> (w1819:bool)
            n1500 = Subtract(x=w1831, y="Mean T1 Position\nto compare (nm)") -> (x-y=w1824:dbl[])
            n1501 = call <vilib>:"Std Deviation and Variance.vi"("X"=w1824) -> ("mean"=→"mean":dbl, "standard deviation"=→"standard\ndeviation":dbl)  [unwired: 1 in, 1 out]
            n1502 = Array Max & Min(array=w1824) -> (max value=→"max value":dbl, min value=→"min value":dbl)  [unwired: 2 out]
            n1503 = Greater?(x=w1824, y="Threshold (nm)") -> (0:w1834:bool[])
            n1504 = case shown="True" w1819 {
              tunnel: w1816 -> [_ w1840]
              tunnel: w1815 -> [_ w1839]
              tunnel: [FALSE ("TTrig?") w1838] -> w1822
              frame False {
              }
              frame True {
                n1505 = xnode "Read/Write Control"("FPGA VI Reference In"=w1840, "error in"=w1839) -> ("TTrig?"=w1838:bool)  [unwired: 2 out]
              }
            }
            n1506 = Or Array Elements(Boolean array=w1834) -> (logical OR=w1821:bool)
            n1507 = Select(t=w1822, s=w1819, f=w1821) -> (s? t:f=w1820:bool)
            n1508 = Not(x=w1819) -> (.not. x?=w1818:bool)
            n1509 = And(x=w1820, y=w1818) -> (x .and. y?=w1817:bool)
            n1510 = Select(t="Triggered", s=w1820, f="Wait for trigger") -> (s? t:f=w1828:string)
            n1511 = case shown="True" w1820 {
              tunnel: [0 0] -> w1827
              tunnel: w1816 -> [_ w1845]
              tunnel: w1815 -> [_ w1844]
              frame False {
                "Waiting" <- TRUE ("Waiting")
              }
              frame True {
                n1512 = xnode "Read/Write Control"("FPGA VI Reference In"=w1845, "error in"=w1844, "TTrig?"=FALSE) -> ()  [unwired: 2 out]
                n1513 = local read "Messages"() -> (w1848:string)
                n1514 = call <vilib>:"Beep.vi"() -> ()  [unwired: 12 in]
                n1515 = call "Update messages.vi"("Message to add"="Unwinding trigger.", "Old message string"=w1848) -> ("New message string"=w1849:string)
                n1516 = local write "Messages"(w1849) -> ()
                n1517 = local write "Waiting"(FALSE ("Waiting")) -> ()
                "Triggered" <- TRUE ("Triggered")
              }
            }
            n1518 = case "Only need to turn on laser if host triggered" shown="True" w1817 {
              frame False {
              }
              frame True {
                n1519 = property on="Green Laser ON/Interlacing" class="Bool (strict)"("Val(Sgnl)"=TRUE ("Value (Signaling)")) -> ()  [unwired: 2 in, 2 out]
              }
            }
          }
          frame "Triggered" {
            n1520 = local read "Trap Trig. (FPGA)"() -> (w1856:bool)
            n1521 = Increment(x=w1859) -> (x+1=w1857:i32)
            n1522 = Greater Or Equal?(x=w1857, y="Fl. ON time (n)") -> (x >= y?=w1855:bool)
            n1523 = Select(t="Wait for trigger", s=w1855, f="Triggered" ("t")) -> (s? t:f=w1860:string)
            n1524 = And(x=w1855, y=w1856) -> (x .and. y?=w1852:bool)
            n1525 = case shown="True" w1852 {
              tunnel: w1854 -> [_ w1864]
              tunnel: w1853 -> [_ w1863]
              frame False {
              }
              frame True {
                n1526 = xnode "Read/Write Control"("FPGA VI Reference In"=w1864, "error in"=w1863, "FPGA Trap Trig"=TRUE) -> ()  [unwired: 2 out]
              }
            }
            n1527 = case shown="True" w1855 {
              frame False {
              }
              frame True {
                w1866 = FALSE ("Value (Signaling)")
                n1528 = local write "Triggered"(w1866) -> ()
                n1529 = local write "Waiting"(TRUE ("Waiting")) -> ()
                n1530 = property on="Green Laser ON/Interlacing" class="Bool (strict)"("Val(Sgnl)"=w1866) -> ()  [unwired: 2 in, 2 out]
              }
            }
          }
          frame "Do nothing" {
          }
          frame "Initialize", Default {
            n1531 = Increment(x=w1877) -> (x+1=w1881:i32)
            n1532 = Select(t=1, s=w1870, f=w1881) -> (s? t:f=w1871:i32)
            n1533 = feedback #27(w1879) -> (w1885:dbl[])
            n1534 = Build Array (concatenate)(w1879, w1885) -> (w1878:dbl[])
            n1535 = Greater Or Equal?(x=w1871, y="Wait to get offset (n)") -> (x >= y?=w1874:bool)
            n1536 = Select(t=w1879, s=w1870, f=w1878) -> (s? t:f=w1880:dbl[])
            n1537 = feedback-in #27(w1880) -> ()
            n1538 = call-poly <vilib>:"Mean.vi"("X"=w1880) -> ("mean"=w1875:dbl)  [unwired: 1 out]
            n1539 = local write "Mean T1 Position\nto compare (nm)"(w1875) -> ()
            n1540 = case shown="True" w1870 {
              tunnel: w1873 -> [_ w1891]
              tunnel: w1872 -> [_ w1890]
              frame False {
              }
              frame True {
                w1887 = FALSE ("FPGA Trap Trig")
                n1541 = xnode "Read/Write Control"("FPGA VI Reference In"=w1891, "error in"=w1890, "FPGA Trap Trig"=w1887) -> ("FPGA VI Reference Out"=w1889:T19, "error out"=w1888:errorcluster)
                n1542 = xnode "Read/Write Control"("FPGA VI Reference In"=w1889, "error in"=w1888, "TTrig?"=w1887) -> ()  [unwired: 2 out]
              }
            }
            n1543 = Select(t="Wait for trigger", s=w1874, f="Initialize") -> (s? t:f=w1882:string)
            n1544 = case shown="True" w1874 {
              tunnel: w1875 -> [_ w1894]
              tunnel: w1873 -> [_ w1903]
              tunnel: w1872 -> [_ w1902]
              frame False {
                n1545 = local write "Waiting"(FALSE ("Waiting")) -> ()
                "Initializing" <- TRUE ("Initializing")
              }
              frame True {
                n1546 = local read "Threshold (nm)"() -> (w1906:dbl)
                n1547 = local read "AOM X Cal (nm/MHz)"() -> (w1905:dbl)
                n1548 = Add(x=w1894, y=w1906) -> (x+y=w1907:dbl)
                n1549 = Divide(x=w1907, y=w1905) -> (x/y=w1904:dbl)
                n1550 = call "IR AOM freq to word.vi"("Frequency In (MHz)"=w1904) -> ("Frequency Word Out (double)"=w1901:dbl)
                n1551 = local write "Initializing"(FALSE ("Initializing")) -> ()
                n1552 = local write "Waiting"(TRUE ("Waiting")) -> ()
                n1553 = To Quad Integer(1:w1901) -> (0:w1900:i64)
                n1554 = xnode "Read/Write Control"("FPGA VI Reference In"=w1903, "error in"=w1902, "FPGA TTrig Thresh"=w1900) -> ("FPGA VI Reference Out"=w1897:T19, "error out"=w1896:errorcluster)
                n1555 = xnode "Read/Write Control"("FPGA VI Reference In"=w1897, "error in"=w1896, "FPGA Trap Trig"=TRUE) -> ()  [unwired: 2 out]
              }
            }
          }
        }
      }
    }
    n1556 = feedback-in #24(w1478) -> ()
    n1557 = feedback-in #25(w1475) -> ()
    n1558 = Split 1D Array(array=w1430, index=w1492) -> (first subarray=w1602:dbl[])  [unwired: 1 out]
    n1559 = feedback-in #26(w1602) -> ()
    n1560 = call-poly <vilib>:"Mean.vi"("X"=w1602) -> ("mean"=w1601:dbl)  [unwired: 1 out]
    "Bead Mean (nm)" <- w1601
    n1561 = Subtract(x=w1602, y=w1601) -> (x-y=w1600:dbl[])
    n1562 = Square(x=w1600) -> (x^2=w1599:dbl[])
    n1563 = call-poly <vilib>:"Mean.vi"("X"=w1599) -> ("mean"=w1598:dbl)  [unwired: 1 out]
    n1564 = Square Root(x=w1598) -> (sqrt(x)=w1597:dbl)
    n1565 = Multiply(x=10.0, y=w1597) -> (x*y=→"RMS (Ang)":dbl)
    n1566 = xnode ("Read/Write Control")("FPGA VI Reference In"=w1635, "error in"=w1634) -> ("FPGA VI Reference Out"=w1460:T19, "error out"=w1459:errorcluster, "AI2 Y Sum Set 1"=w1741:i16, "AI2 Y Sum Set 2"=w1740:i16, "AI1 X Set 1"=w1524:fxp<+/-,16,1>, "AI1 X Set 2"=w1523:fxp<+/-,16,1>, "Trap Pos FB Int Signal"=→"Trap Pos FB Int Signal":fxp<+/-,24,9>, "Trap Pos FB Int-Norm Signal"=→"Trap Pos FB Int-Norm Signal":fxp<+/-,16,1>, "Trap Pos FB Action"=w1517:i64, "Scanning"=→"AOD Scanning":bool, "Scan I"=→"AOD Scan I":u64, "Scanning MCL"=w1743:bool, "Scan I (MCL)"=→"MCL Scan I":u64, "Green FB Signals"=w1680:T43, "Trap Pos FB Action"=w1447:i64, "TTrig Fin Thresh"=w1443:i64)
    "MCL Scanning" <- w1743
    "Trap Pos FB Action" <- w1517
    n1567 = local read "FB Trig Integrate"() -> (w1441:u32)
    n1568 = Divide(x=w1447, y=w1441) -> (x/y=w1440:dbl)
    "TTrig Sig (Int)" <- w1440
    n1569 = Divide(x=w1443, y=w1441) -> (x/y=w1438:dbl)
    "TTrig Fin Thresh (Int)" <- w1438
    n1570 = local read "AOM X Cal (nm/MHz)"() -> (w1446:dbl)
    n1571 = local read "AI2 (V)"() -> (w1742:cluster{"Set 1":dbl, "Set 2":dbl})
    n1572 = Bundle By Name(cluster=w1742, "Set 1"=w1741, "Set 2"=w1740) -> (w1738:cluster{"Set 1":dbl, "Set 2":dbl})
    n1573 = Divide(x=w1517, y=327.67) -> (x/y=→"Action (%)":dbl)
    n1574 = local read "Trap X (AI1)"() -> (w1537:T10)
    n1575 = call "IR AOM word double to freq.vi"("Frequency Word In (double)"=w1438) -> ("Frequency Out (MHz)"=w1437:dbl)
    n1576 = call "IR AOM word double to freq.vi"("Frequency Word In (double)"=w1440) -> ("Frequency Out (MHz)"=w1439:dbl)
    n1577 = Divide(x=w1738, y=3276.7) -> (x/y=w1737:cluster{"Set 1":dbl, "Set 2":dbl})
    n1578 = Multiply(x=w1439, y=w1446) -> (x*y=w1445:dbl)
    "TTrig Sig (nm)" <- w1445
    n1579 = Multiply(x=w1437, y=w1446) -> (x*y=w1444:dbl)
    "TTrig Fin Thresh (nm)" <- w1444
    n1580 = local write "AI2 (V)"(w1737) -> ()
    n1581 = Bundle(cluster=w1537, "Trap 1"=w1524, "Trap 2"=w1523) -> (→"Trap X (AI1)":T10)
    n1582 = Bundle(w1445, w1444) -> (→"TTrig":cluster{dbl, dbl})  [unwired: 1 in]
    n1583 = Divide(x=w1680, y=3276.7) -> (x/y=w1676:T44)
    n1584 = Unbundle By Name(w1676) -> ("Green FB Ch 0"=w1679:dbl, "Green FB Ch 1"=w1678:dbl, "Green FB Ch 2"=w1677:dbl)
    n1585 = Divide(x=w1679, y=w1677) -> (x/y=w1675:dbl)
    n1586 = Divide(x=w1678, y=w1677) -> (x/y=w1674:dbl)
    n1587 = flat-sequence "To save data" {
      tunnel: [w2762] -> w1761
      tunnel: [w2763] -> w1760
      tunnel: w1711 -> [w2756]
      tunnel: w1465 -> [w2760]
      tunnel: ["Save Calibration"] -> w1734
      tunnel: w1731 -> [w2759]
      tunnel: [w2752] -> w1730
      tunnel: [w2749] -> w1729
      tunnel: [w2746] -> w1728
      tunnel: w1710 -> [w2748]
      tunnel: w1617 -> [w2742]
      tunnel: [w2742] -> w1616
      tunnel: ["Start Saving"] -> w1582
      tunnel: [w2736] -> w1505
      tunnel: [w2735] -> w1504
      tunnel: w1761 -> [w2998]
      tunnel: w1760 -> [w2997]
      tunnel: w1506 -> [w2996]
      tunnel: w1734 -> [w2995]
      tunnel: w1730 -> [w2993]
      tunnel: w1729 -> [w2992]
      tunnel: w1728 -> [w2991]
      tunnel: w1591 -> [w2990]
      tunnel: w1627 -> [w2989]
      tunnel: w1616 -> [w2988]
      tunnel: w1582 -> [w2987]
      tunnel: w1580 -> [w2986]
      tunnel: w1556 -> [w2985]
      tunnel: w1505 -> [w2984]
      tunnel: w1504 -> [w2983]
      tunnel: w1503 -> [w2982]
      tunnel: w1426 -> [w2981]
      frame #0 {
        n1588 = Or(x="Save N Sets", y="Start Saving") -> (x .or. y?=w2743:bool)
        n1589 = To Double Precision Float(number=w2759) -> (double precision float=w2753:dbl)
        n1590 = Build Array(w2743, "Save Calibration", w2756, w2748) -> (w2758:bool[])
        n1591 = Compound Arithmetic op=OR("Save Calibration", w2756, w2743, w2748) -> (w2761:bool)
        n1592 = Boolean Array To Number(Boolean array=w2758) -> (number=w2755:u32)
        n1593 = feedback #28(FALSE ("Save APD Data\nwith Trap Data")) -> (w2737:bool)
        n1594 = feedback #29(refnum<k0> refnum) -> (w2764:refnum<file>)
        n1595 = feedback #30(refnum<k0> refnum) -> (w2739:refnum<file>)
        n1596 = feedback #31(FALSE ("Save APD Data\nwith Trap Data")) -> (w2747:bool)
        n1597 = feedback #32(refnum<k0> refnum) -> (w2750:refnum<file>)
        n1598 = feedback #33(0) -> (w2766:i32)
